vi "Saturn SPI Addr Calc.vi"() -> ()   [LabVIEW 2009]
panel:
  in  "stop":bool
  out "d1 2":u16
  out "0x1 2":u16 format="%04x"
  out "d1":u16
  out "0x1":u16 format="%04x"
  in  "Saturn Base Addresses":u16(ring)=64 items=["PH1"=64, "PH2"=128, "PH3"=192, "PH4"=256, "PH5"=320, "PH6"=384, "PH7"=448, "PH8"=512, "PH9"=576, "PH10"=640, "PH11"=704, "PH12"=768, "PH13"=832, "PH14"=896, "PH15"=960, "PH16"=1024, "PH17"=1088, "PH18"=1152, "PH19"=1216, "PH20"=1280, "PH21"=1344, "PH22"=1408, "PH23"=1472, "PH24"=1536, "RAM1"=2048, "RAM2"=2304]
  in  "Saturn PHASE Reg Offsets":T1(ring)
  in  "Saturn CTL Registers":T2(ring)
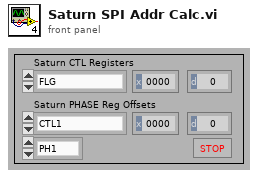
[diagram p1: front panel]
types:
  T1 = enum16{"CTL1", "CTL2", "STPA", "STBB", "STBC", "OFST", "DLYL", "DLYU", "CDIV", "AMP1L", "AMP1U", "AMP2L", "AMP2U", "AMP3L", "AMP3U", "AMP4L", "AMP4U", "AMP5L", "AMP5U", "AMP6L", "AMP6U", "AMP7L", "AMP7U", "AMP8L", "AMP8U", "AMP9L", "AMP9U", "AMP10L", "AMP10U", "AMP11L", "AMP11U", "AMP12L", "AMP12U", "AMP13L", "AMP13U", "AMP14L", "AMP14U", "AMP15L", "AMP15U", "AMP16L", "AMP16U", "AMP17L", "AMP17U", "AMP18L", "AMP18U", "AMP19L", "AMP19U", "AMP20L", "AMP20U", "AMP21L", "AMP21U", "AMP22L", "AMP22U", "AMP23L", "AMP23U", "AMP24L", "AMP24U", "AMP25L", "AMP25U", "AMP26L", "AMP26U", "PG_TIMEOUT", "RESERVED_1", "RESERVED_2"}
  T2 = enum16{"FLG", "ENABLE", "WE1", "WE2", "WE3", "WE4", "WE5", "RVLD1", "RVLD2", "RVLD3", "RVLD4", "RVLD5", "SEQ0A", "SEQ0B", "SEQ1A", "SEQ1B", "RECT1", "RECT2", "RECT3", "RECT4", "RECT5", "RECT6", "CIM0", "CIM1", "CIM_GCL", "CIM_GCU", "SH_PHASE", "SH_DELAYL", "SH_DELAYU", "HV_CTRL", "CM_CTRL", "VG_CTRL", "BC_CTRL0", "BC_CTRL1", "BG_CTRL", "PGO_CTRL", "CG_CTRL", "WFD_CTRL", "ACCA", "ACCB", "ACCC", "WDAC", "SEQSTATE", "CPH", "TESTEN", "TESTSEL", "ATSTCTRL0", "ATSTCTRL1", "ATSTCTRL2", "ATSTCTRL3", "ATSTCTRL4"}
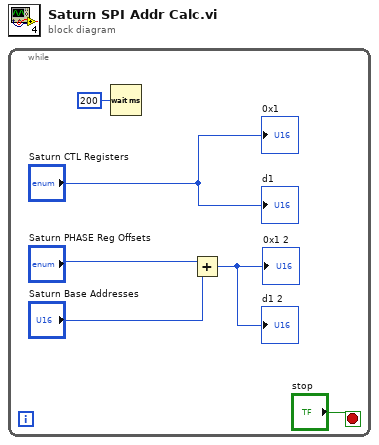
[diagram p0: block diagram]
diagram:
  n1 = while {
    stop <- "stop" stop-if-true
    n2 = Wait (ms)(milliseconds to wait=u32 200) -> ()  [unwired: 1 out]
    n3 = Add(x="Saturn PHASE Reg Offsets", y="Saturn Base Addresses") -> (x+y=→"0x1 2" →"d1 2":u16)
    "0x1" <- "Saturn CTL Registers"
    "d1" <- "Saturn CTL Registers"
  }
